vi "Create Signature String.vi"(10 "HTTP Session in":refnum<class "Session.lvclass">) -> (2 "Encoded signature":string, 3 "HTTP Session out":refnum<class "Session.lvclass">)   [LabVIEW 2015, in "NI_Azure_Core.lvlib" / "Session.lvclass"]
uses:
  Session.lvclass
  Session.lvclass/Session.ctl
  Read Access Key.vi
  Read HTTP Verb.vi
  Read Signature Fields.vi
  Read Content Length.vi
  NI_Azure_Core.lvlib
  <vilib>/httpClient/LabVIEWHTTPClient.lvlib
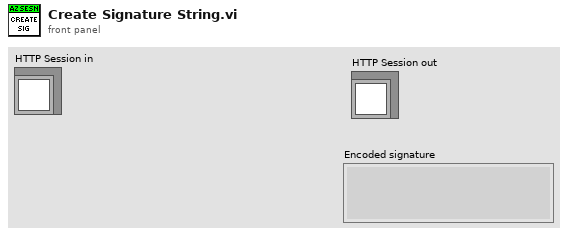
[diagram p1: front panel]
types:
  T1 = typedef "NI_Azure_Core.lvlib/Session.lvclass/Signature Fields.ctl" = cluster{"Content-Encoding":string, "Content-Language":string, "Content-Length":string, "Content-MD5":string, "Content-Type":string, "Date":string, "If-Modified-Since":string, "If-Match":string, "If-None-Match":string, "If-Unmodified-Since":string, "Range":string}
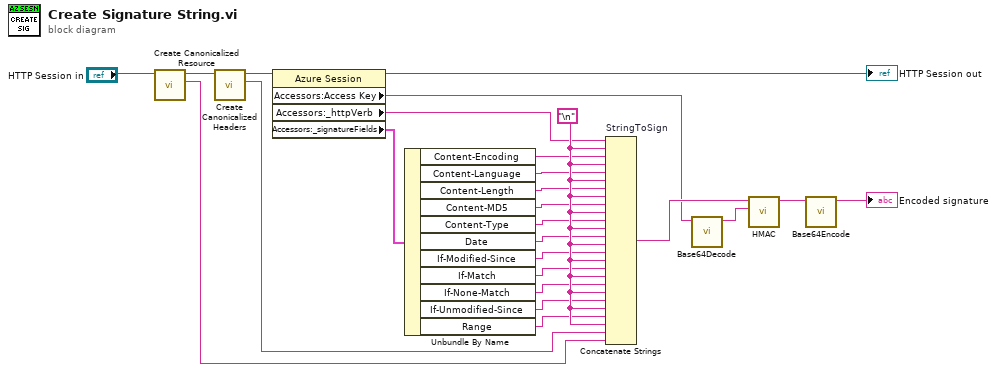
[diagram p0: block diagram]
diagram:
  w21 = "\n"
  n1 = call "Create Canonicalized Resource.vi"("HTTP Session in"="HTTP Session in") -> ("Canonical resource"=w1:string, "HTTP Session out"=w2:refnum<class "Session.lvclass">)  [unwired: 8 in]
  n2 = call "Create Canonicalized Headers.vi"("HTTP Session in"=w2) -> ("Canonical headers"=w4:string, "HTTP Session out"=w5:refnum<class "Session.lvclass">)  [unwired: 8 in]
  n3 = property class="Azure Session"(reference=w5) -> (reference out=→"HTTP Session out":refnum<class "Session.lvclass">, "Accessors:Access Key"=w19:string, "Accessors:_httpVerb"=w6:string, "Accessors:_signatureFields"=w18:T1)  [unwired: 1 in, 1 out]
  n4 = Unbundle By Name(w18) -> ("Content-Encoding"=w17:string, "Content-Language"=w16:string, "Content-Length"=w7:string, "Content-MD5"=w15:string, "Content-Type"=w14:string, "Date"=w13:string, "If-Modified-Since"=w12:string, "If-Match"=w11:string, "If-None-Match"=w10:string, "If-Unmodified-Since"=w9:string, "Range"=w8:string)
  n5 = Concatenate Strings "StringToSign"(w6, w21, w17, w21, w16, w21, w7, w21, w15, w21, w14, w21, w13, w21, w12, w21, w11, w21, w10, w21, w9, w21, w8, w21, w4, w1) -> (w24:string)
  n6 = call <vilib>:"Base64Decode.vi"("buffer in"=w19) -> ("decoded string"=w23:string)  [unwired: 9 in, 1 out]
  n7 = call "HMAC.vi"("Key"=w23, "Message"=w24) -> ("Keyed Hash"=w22:string)  [unwired: 9 in]
  n8 = call <vilib>:"Base64Encode.vi"("buffer in"=w22) -> ("encoded string"=→"Encoded signature":string)  [unwired: 9 in, 1 out]
